vi "WriteSimpleLogFile.vi"(9 "StartTime":string, 10 "Status":string, 11 "SerialNumber":string) -> (3 "#OfTest":string)   [LabVIEW 2018]
uses:
  <vilib>/Utility/file.llb/Write To Spreadsheet File (string).vi
panel:
  out "TestStatusArray":string[](array[string])
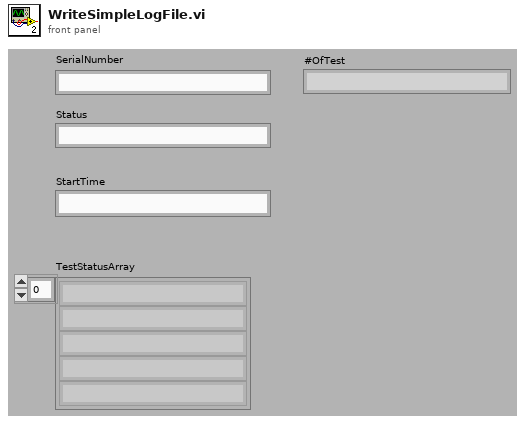
[diagram p1: front panel]
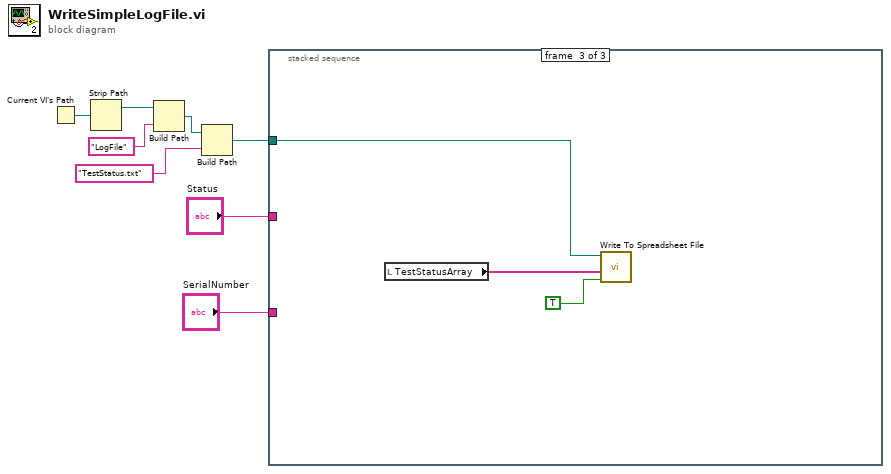
[diagram p0: block diagram]
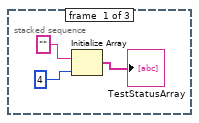
[diagram p2: hidden frame]
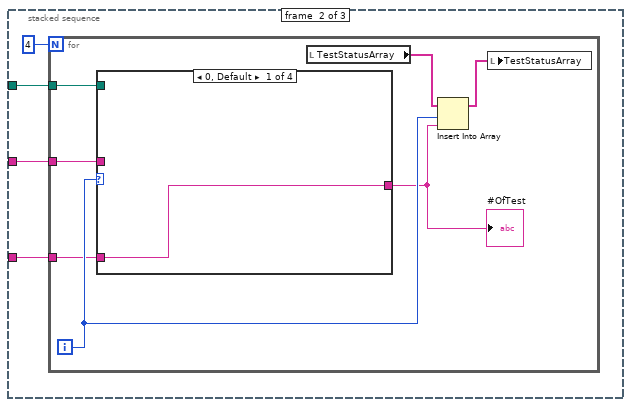
[diagram p3: hidden frame]
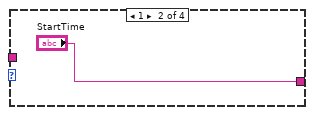
[diagram p4: hidden frame]
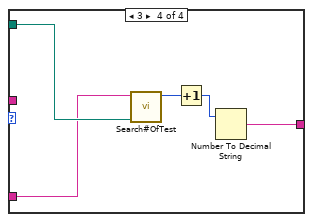
[diagram p6: hidden frame]
diagram:
  n1 = Current VI's Path() -> (path=w8:path)
  n2 = Strip Path(path=w8) -> (stripped path=w7:path)  [unwired: 1 out]
  n3 = Build Path(base path=w7, name or relative path="LogFile") -> (appended path=w5:path)
  n4 = Build Path(base path=w5, name or relative path="TestStatus.txt") -> (appended path=w3:path)
  n5 = stacked-sequence {
    tunnel: "Status" -> [_ w14 _]
    tunnel: w3 -> [_ w13 w31]
    tunnel: "SerialNumber" -> [_ w12 _]
    frame #0 {
      n6 = Initialize Array("", 4 ("dimension size")) -> (→"TestStatusArray":string[])
    }
    frame #1 {
      n7 = for {
        N: 4 -> [_]
        tunnel: w14 -> [w18]
        tunnel: w13 -> [w17]
        tunnel: w12 -> [w16]
        i -> [w20]
        n8 = case shown="0, Default" w20 {
          tunnel: [w23 "StartTime" w25 w28] -> w19
          tunnel: w18 -> [_ _ w25 _]
          tunnel: w17 -> [_ _ _ w27]
          tunnel: w16 -> [w23 _ _ w26]
          frame 0, Default {
          }
          frame 1 {
          }
          frame 2 {
          }
          frame 3 {
            n9 = call "Search#OfTest.vi"("TestStatusPath"=w27, "MatchedSerialNumber"=w26) -> ("#OfTest"=w30:i32)  [unwired: 9 out]
            n10 = Increment(x=w30) -> (x+1=w29:i32)
            n11 = Number To Decimal String(number=w29) -> (decimal integer string=w28:string)  [unwired: 1 out]
          }
        }
        "#OfTest" <- w19
        n12 = local read "TestStatusArray"() -> (w22:string[])
        n13 = Insert Into Array(array=w22, index=w20, new element=w19) -> (w21:string[])
        n14 = local write "TestStatusArray"(w21) -> ()
      }
    }
    frame #2 {
      n15 = local read "TestStatusArray"() -> (w32:string[])
      n16 = call-poly <vilib>:"Write To Spreadsheet File.vi"("append to file? (new file:F)"=TRUE, "1D data"=w32, "file path (dialog if empty)"=w31) -> ()  [unwired: 3 in, 3 out]
    }
  }
